vi "test_VI Set_Get Protocol TCP.vi"(8 "error in (no error)":errorcluster, 11 "TestCase in":refnum<class "Instrument Addon Scripting API Custom Device Unit Tests.lvclass">) -> (0 "error out":errorcluster, 3 "TestCase out":refnum<class "Instrument Addon Scripting API Custom Device Unit Tests.lvclass">)   [LabVIEW 2018, in "Instrument Addon Scripting API Custom Device Unit Tests.lvclass"]
uses:
  Instrument Addon Scripting API Custom Device Unit Tests.lvclass
  Addon/Support Libraries/Protocols.lvlibp/TCP/TCP.lvclass
  C:/Users/nitest/Git/NI VS Instrument Addon Fork/Source/Addon/Support Libraries/Protocols.lvlibp/Protocol Parent/Protocol Parent.lvclass
  NationalInstruments.VeriStand.SystemDefinitionAPI
  Addon/Support Libraries/Protocols.lvlibp/TCP/Data Access/Write IP Address.vi
  Addon/Support Libraries/Protocols.lvlibp/TCP/Data Access/Write Port.vi
  Instrument Addon Scripting API Test Assets/Instrument Addon Scripting API Test Assets.lvclass
  <vilib>/addons/_JKI Toolkits/VI Tester/TestCase.llb/TestCase.lvclass
  APIs/Scripting API/Instrument Addon Scripting API.lvlib
  C:/Program Files (x86)/National Instruments/LabVIEW 2018/vi.lib/addons/_JKI Toolkits/VI Tester/TestCase.llb/TestCase.lvclass
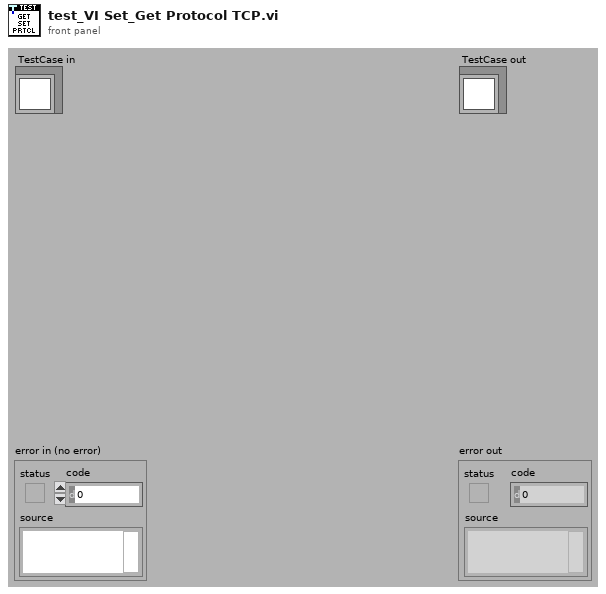
[diagram p1: front panel]
types:
  T1 = typedef "Custom Device API.lvlib/Custom Device Item Ref.ctl" = u64
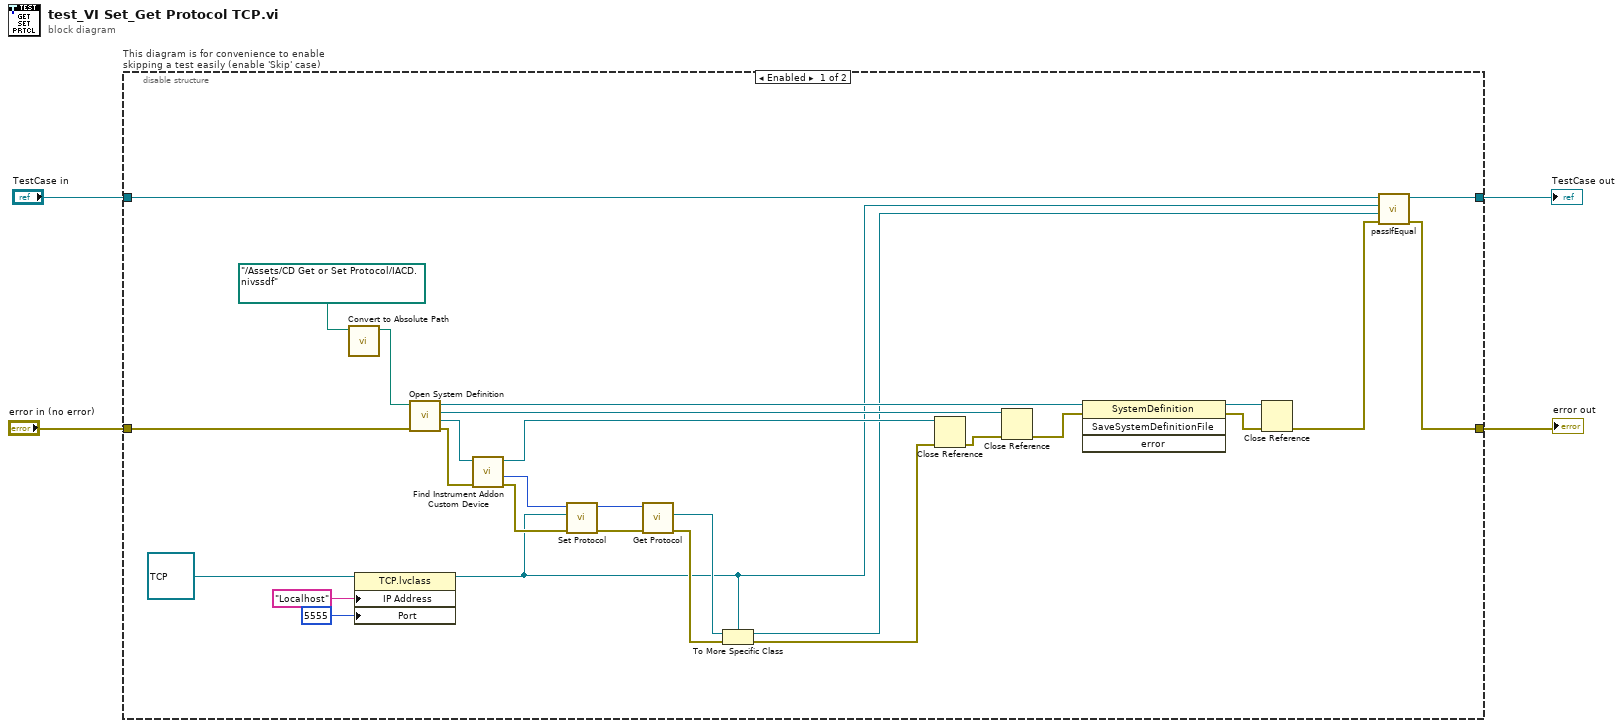
[diagram p0: block diagram]
diagram:
  n1 = disable-structure "This diagram is for convenience to enable skipping a test easily (enable 'Skip' case)" shown="Enabled" {
    disable-tunnel: "TestCase in" -> [w13 w36]
    disable-tunnel: [w12 w34] -> w1
    disable-tunnel: [w8 w35] -> w3
    disable-tunnel: "error in (no error)" -> [w32 w33]
    frame Enabled {
      n2 = call "Convert to Absolute Path.vi"("System Definition File"=path "../Assets/CD Get or Set Protocol/IACD.nivssdf" ("SDF file")) -> ("Absolute Path"=w30:path)  [unwired: 10 in]
      n3 = property class="TCP.lvclass"(reference=refnum<class "TCP.lvclass"> refnum ("Protocols.lvlibp:TCP.lvclass"), "IP Address"="Localhost" ("VISA Resource"), "Port"=u16 5555 ("Local Port")) -> (reference out=w10:refnum<class "TCP.lvclass">)  [unwired: 1 in, 1 out]
      n4 = call "Open System Definition.vi"("error in (no error)"=w32, "System Definition File"=w30) -> ("error out"=w27:errorcluster, "Target Refnum"=w26:refnum<k24>, "Root Refnum"=w29:refnum<k24>, "System Definition Refnum"=w20:refnum<k24>)  [unwired: 6 in]
      n5 = call "Find Instrument Addon Custom Device.vi"("error in"=w27, "target in"=w26) -> ("error out"=w25:errorcluster, "NodeID"=w24:u64, "target out"=w23:refnum<k24>)  [unwired: 7 in]
      n6 = call "Set Protocol.vi"("Error In"=w25, "Protocol in"=w10, "Instrument Addon Refnum In"=w24) -> ("Error Out"=w21:errorcluster, "Instrument Addon Refnum Out"=w22:T1)  [unwired: 7 in]
      n7 = call "Get Protocol.vi"("Error In"=w21, "Instrument Addon Refnum In"=w22) -> ("Error Out"=w15:errorcluster, "Protocol"=w16:refnum<class "Protocol Parent.lvclass">)  [unwired: 7 in, 1 out]
      n8 = To More Specific Class(target class=w10, reference=w16, error in=w15) -> (specific class reference=w11:refnum<class "TCP.lvclass">, error out=w14:errorcluster)
      n9 = Close Reference(reference=w23, error in (no error)=w14) -> (error out=w28:errorcluster)
      n10 = Close Reference(reference=w29, error in (no error)=w28) -> (error out=w19:errorcluster)
      n11 = invoke class="SystemDefinition" method="SaveSystemDefinitionFile"(reference=w20, error in=w19) -> (reference out=w18:refnum<k24>, error out=w17:errorcluster)  [unwired: 2 in, 2 out]
      n12 = Close Reference(reference=w18, error in (no error)=w17) -> (error out=w9:errorcluster)
      n13 = call-dynamic "passIfEqual.vi"("error in (no error)"=w9, "y"=w11, "x"=w10, "TestCase in"=w13) -> ("error out"=w8:errorcluster, "TestCase out"=w12:refnum<class "Instrument Addon Scripting API Custom Device Unit Tests.lvclass">)  [unwired: 6 in]
    }
    frame Disabled {
      # "skip test result while test is under development"
      n14 = call <vilib>:"skip.vi"("error in (no error)"=w33, "TestCase in"=w36) -> ("error out"=w35:errorcluster, "TestCase out"=w34:refnum<class "Instrument Addon Scripting API Custom Device Unit Tests.lvclass">)  [unwired: 8 in]
    }
  }
  "error out" <- w3
  "TestCase out" <- w1
